vi "Start_MischerMonitor.vi"() -> ()   [LabVIEW 2018]
panel:
  in  "VI-Pfad":path=path "E:/CryoTUM-Software/16T-Magnet_Ultimate-Control_Version_2-0/LS370Monitor.vi"
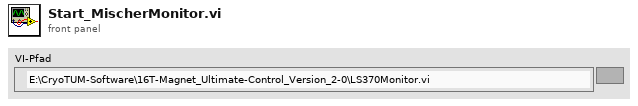
[diagram p1: front panel]
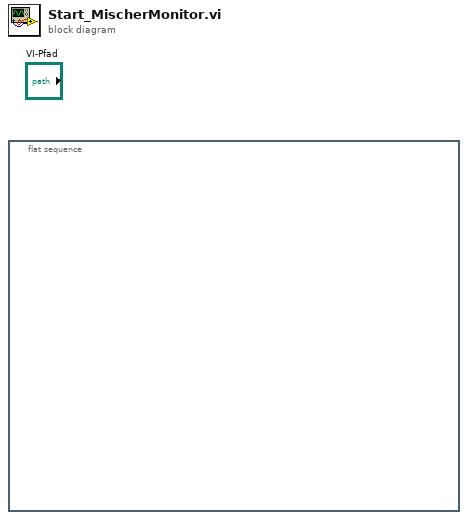
[diagram p0: block diagram]
diagram:
  n1 = flat-sequence {
    frame #0 {
    }
  }
